vi "Send Que Notifier Final Working.vi"() -> ()   [LabVIEW 2022 SP3]
panel:
  in  "stop":bool
  in  "error in (no error)":errorcluster
  out "error out":errorcluster
  out "Sent Que":i32[](array[numeric])
  out "Sent Notifier":u8
  in  "Que Send":bool
  in  "Nitification Send":bool
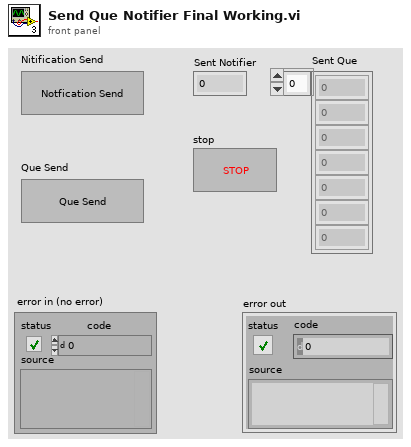
[diagram p1: front panel]
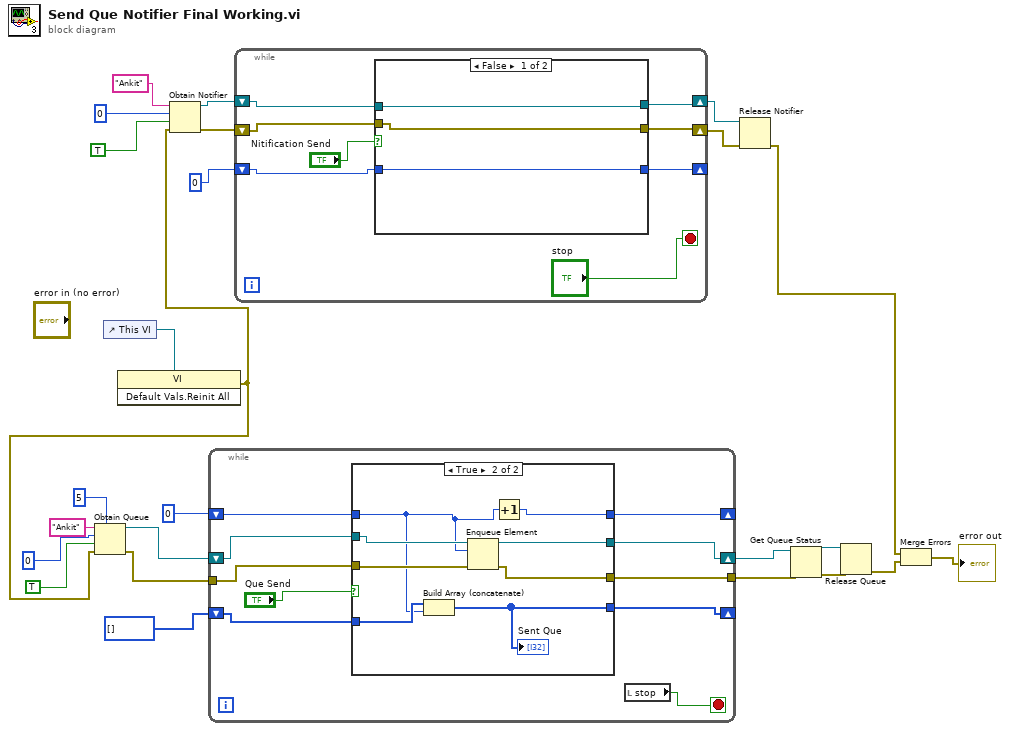
[diagram p0: block diagram]
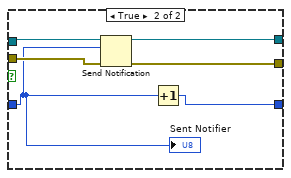
[diagram p3: hidden frame]
diagram:
  n1 = control-ref of="This VI"() -> (w19:refnum<vi>)
  n2 = invoke class="VI" method="Default Vals.Reinit All"(reference=w19) -> (error out=w11:errorcluster)  [unwired: 2 in, 2 out]
  n3 = Obtain Queue(max queue size (-1, unlimited)=5, name (unnamed)="Ankit", element data type=0 ("max queue size (-1, unlimited)"), create if not found? (T)=TRUE, error in (no error)=w11) -> (queue out=w12:refnum<queue>, error out=w9:errorcluster)  [unwired: 1 out]
  n4 = Obtain Notifier(name (unnamed)="Ankit", notification data type=0, create if not found? (T)=TRUE, error in (no error)=w11) -> (notifier out=w25:refnum<notifier>, error out=w24:errorcluster)  [unwired: 1 out]
  n5 = while {
    shift-right: [w27] -> _
    shift-left: 0 -> [w32]
    shift-right: [w28] -> w7
    shift-left: w12 -> [w31]
    shift-right: [w26] -> _
    shift-left: i32[] [] -> [w33]
    tunnel: w9 -> [w30]
    tunnel: [w29] -> w6
    stop <- w35 stop-if-true
    n6 = case shown="True" "Que Send" {
      tunnel: w33 -> [w36 w42]
      tunnel: w32 -> [w39 w41]
      tunnel: w31 -> [w38 w47]
      tunnel: w30 -> [w37 w46]
      tunnel: [w37 w45] -> w29
      tunnel: [w38 w44] -> w28
      tunnel: [w39 w43] -> w27
      tunnel: [w36 w40] -> w26
      frame False {
      }
      frame True {
        n7 = Build Array (concatenate)(w42, w41) -> (w40:i32[])
        "Sent Que" <- w40
        n8 = Enqueue Element(queue=w47, element=w41, error in (no error)=w46) -> (queue out=w44:refnum<queue>, error out=w45:errorcluster)  [unwired: 1 in, 1 out]
        n9 = Increment(x=w41) -> (x+1=w43:i32)
      }
    }
    n10 = local read "stop"() -> (w35:bool)
  }
  n11 = while {
    shift-right: [w52] -> w21
    shift-left: w25 -> [w54]
    shift-right: [w51] -> w20
    shift-left: w24 -> [w53]
    shift-right: [w49] -> _
    shift-left: 0 -> [w50]
    stop <- "stop" stop-if-true
    n12 = case shown="False" "Nitification Send" {
      tunnel: w54 -> [w58 w64]
      tunnel: w53 -> [w57 w63]
      tunnel: [w58 w62] -> w52
      tunnel: [w57 w61] -> w51
      tunnel: w50 -> [w56 w60]
      tunnel: [w56 w59] -> w49
      frame False {
      }
      frame True {
        n13 = Send Notification(notification=w60, notifier=w64, error in (no error)=w63) -> (notifier out=w62:refnum<notifier>, error out=w61:errorcluster)
        n14 = Increment(x=w60) -> (x+1=w59:i32)
        "Sent Notifier" <- w60
      }
    }
  }
  n15 = Release Notifier(notifier=w21, error in (no error)=w20) -> (error out=w3:errorcluster)  [unwired: 1 in, 2 out]
  n16 = Get Queue Status(queue=w7, error in (no error)=w6) -> (queue out=w4:refnum<queue>, error out=w5:errorcluster)  [unwired: 1 in, 6 out]
  n17 = Release Queue(queue=w4, error in (no error)=w5) -> (error out=w1:errorcluster)  [unwired: 1 in, 2 out]
  n18 = Merge Errors(w3, w1) -> (→"error out":errorcluster)
